vi "例4-28.vi"() -> ()   [LabVIEW 2019]
panel:
  in  "停止":bool
  out "报警灯":bool
  out "温度":dbl format="%#_4g"
  out "波形图表":dbl(graph)
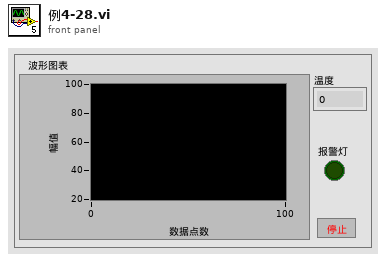
[diagram p1: front panel]
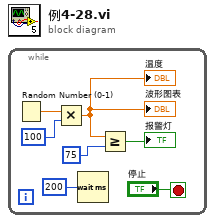
[diagram p0: block diagram]
diagram:
  n1 = while {
    stop <- "停止" stop-if-true
    n2 = Random Number (0-1)() -> (number: 0 to 1=w7:dbl)
    n3 = Multiply(x=w7, y=100) -> (x*y=w4:dbl)
    "波形图表" <- w4
    "温度" <- w4
    n4 = Wait (ms)(milliseconds to wait=200) -> ()  [unwired: 1 out]
    n5 = Greater Or Equal?(x=w4, y=75) -> (x >= y?=→"报警灯":bool)
  }
